vi "while loop break_0.vi"() -> ()   [LabVIEW 2015]
panel:
  in  "Tab Control":enum32{"Page 1", "Page 2"}(tab)
  in  "While loop break":i32
  out "While loop counter":i32
  # "While loop Break"
  # "Pardeep Kumar"
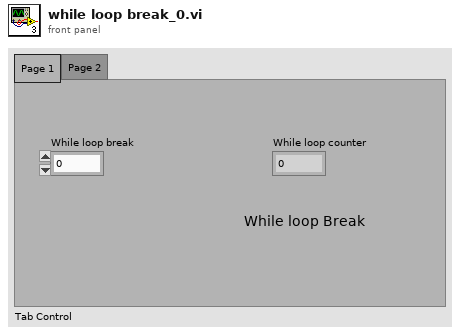
[diagram p1: front panel]
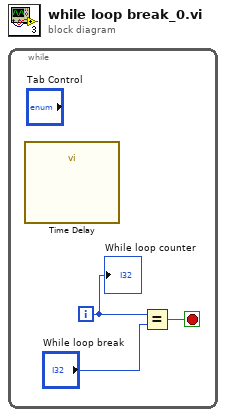
[diagram p0: block diagram]
diagram:
  n1 = while {
    i -> [w3]
    stop <- w1 stop-if-true
    n2 = call "Time Delay"() -> ()  [unwired: 11 in, 1 out]
    n3 = Equal?(x=w3, y="While loop break") -> (x = y?=w1:bool)
    "While loop counter" <- w3
  }
